vi "HEWH Spec Data.vi"(5 "Water Heater Type":T7, 7 "Test Type":T1, 8 "error in (no error)":errorcluster, 11 "UEF Calculated Values Input":T2 {"Data Indexes"."15 sec after Draw Index" format="%#.2f"; "Data Indexes"."15 sec after Draw Timestamp" format="%#.2f"; "Data Indexes"."Test Start Timestamp" format="%.2f"; "Data Indexes"."Test End Timestamp" format="%.2f"; "Data Indexes"."T0 Timestamp" format="%.2f"; "Data Indexes"."Tsf Timestamp" format="%.2f"; "Data Indexes"."Tsu0 Timestamp" format="%.2f"; "Data Indexes"."Tmax1 Timestamp" format="%.2f"; "Data Indexes"."Draw Index Timestamp" format="%#.2f"; "Data Indexes"."Non-Draw Timestamp" format="%#.2f"; "Data Indexes"."Heating Timestamp" format="%#.2f"; "Data Indexes"."Start Energy (BTU-Gas)" format="%.6f"; "Data Indexes"."Start Watt Hours" format="%.6f"; "Static Data"."V - Volume of Wh (True)" format="%.5f"; "Static Data"."T-Ambinet Nominal (°F)" format="%.5f"; "Static Data"."T-Inlet Setpoint (°F)" format="%.5f"; "Static Data"."T-Wh Setpoint (°F)" format="%.5f"; "Sampled Data"."Qe (Wh)" format="%.5f"; "Sampled Data"."Tau stby2 (hr)" format="%.5f"; "Sampled Data"."Tastby2 (°F)" format="%.5f"; "Sampled Data"."Qf (BTU)" format="%.5f"; "Sampled Data"."Qe (BTU)" format="%.5f"; "Sampled Data"."Tmax1 (°F)" format="%.5f"; "Sampled Data"."T0 (°F)" format="%.5f"; "Sampled Data"."Qr (BTU)" format="%.5f"; "Sampled Data"."T 24(°F)" format="%.5f"; "Sampled Data"."T astby(°F)" format="%.5f"; "Sampled Data"."T tstby(°F)" format="%.5f"; "Sampled Data"."T su0(°F)" format="%.5f"; "Sampled Data"."T suf(°F)" format="%.5f"; "Sampled Data"."Tau stby_1 (hr)" format="%.5f"; "Sampled Data"."Qsuf (BTU)" format="%.5f"; "Sampled Data"."Qsu0 (BTU)" format="%.5f"; "Calculated Values"."Draw Bonus Volume (gal)" format="%.6f"; "Calculated Values"."Adjustment Factor" format="%.6f"; "Calculated Values"."T*avg_del(n-1)" format="%.6f"; "Calculated Values"."T*min(n-1)" format="%.6f"; "Calculated Values"."T*avg_del(n)" format="%.6f"; "Calculated Values"."Vn" format="%.6f"; "Calculated Values"."Qdm (BTU)" format="%.6f"; "Calculated Values"."QHWD (BTU)" format="%.6f"; "Calculated Values"."QHW (BTU)" format="%.6f"; "Calculated Values"."UEF" format="%.6f"; "Calculated Values"."QHW67 (BTU)" format="%.6f"; "Calculated Values"."Qda (BTU)" format="%.6f"; "Calculated Values"."Qd (BTU)" format="%.6f"; "Calculated Values"."Q (BTU)" format="%.6f"; "Calculated Values"."UA (BTU/(hr*F))" format="%.6f"; "Calculated Values"."Qhr (BTU/hr)" format="%.6f"; "Calculated Values"."Qstby (BTU)" format="%.6f"; "Calculated Values"."nu_r" format="%.6f"; "Calculated Values"."CpUEF (BTU/(lb*F))" format="%.6f"; "Calculated Values"."rho_nu (lb/gal)" format="%.6f"; "Calculated Values"."V1- Vol (Gal)" format="%.6f"; "Calculated Values"."M cluster mass removed (lb)" format="%.6f"; "Calculated Values"."Cp theoretical (BTU/(lbm °F))" format="%.6f"; "Calculated Values"."Tin1 - Mean Inlet 1st Cluster (°F)" format="%.6f"; "Calculated Values"."Tdel1-Mean Outlet 1st Cluster(°F)" format="%.6f"; "Calculated Values"."Cp 24 (BTU/(lb*F))" format="%.6f"; "Calculated Values"."Cp standby (BTU/(lb*F))" format="%.6f"; "Calculated Values"."Cp2 (BTU/(lb*F))" format="%.6f"; "Calculated Values"."Cp1 (BTU/(lb*F))" format="%.6f"; "Calculated Values"."rho 24 (lb/gal)" format="%.6f"; "Calculated Values"."rho standby (lb/gal)" format="%.6f"; "Calculated Values"."rho 2 (lb/gal)" format="%.6f"; "Calculated Values"."Density of cold water All (lbm/gal)" format="%#.3g"; "Calculated Values"."CpHW (BTU/(lbm °F))" format="%#.3g"; "Calculated Values"."Density of hot water All (lbm/gal)" format="%#.3g"; "Calculated Values"."Mass of water All (lbm)" format="%#.3f"}) -> (0 "error out":errorcluster, 3 "UEF Calculated Values Output":T2 {"Data Indexes"."15 sec after Draw Index" format="%#.2f"; "Data Indexes"."15 sec after Draw Timestamp" format="%#.2f"; "Data Indexes"."Test Start Timestamp" format="%.2f"; "Data Indexes"."Test End Timestamp" format="%.2f"; "Data Indexes"."T0 Timestamp" format="%.2f"; "Data Indexes"."Tsf Timestamp" format="%.2f"; "Data Indexes"."Tsu0 Timestamp" format="%.2f"; "Data Indexes"."Tmax1 Timestamp" format="%.2f"; "Data Indexes"."Draw Index Timestamp" format="%#.2f"; "Data Indexes"."Non-Draw Timestamp" format="%#.2f"; "Data Indexes"."Heating Timestamp" format="%#.2f"; "Data Indexes"."Start Energy (BTU-Gas)" format="%.6f"; "Data Indexes"."Start Watt Hours" format="%.6f"; "Static Data"."V - Volume of Wh (True)" format="%.5f"; "Static Data"."T-Ambinet Nominal (°F)" format="%.5f"; "Static Data"."T-Inlet Setpoint (°F)" format="%.5f"; "Static Data"."T-Wh Setpoint (°F)" format="%.5f"; "Sampled Data"."Qe (Wh)" format="%.5f"; "Sampled Data"."Tau stby2 (hr)" format="%.5f"; "Sampled Data"."Tastby2 (°F)" format="%.5f"; "Sampled Data"."Qf (BTU)" format="%.5f"; "Sampled Data"."Qe (BTU)" format="%.5f"; "Sampled Data"."Tmax1 (°F)" format="%.5f"; "Sampled Data"."T0 (°F)" format="%.5f"; "Sampled Data"."Qr (BTU)" format="%.5f"; "Sampled Data"."T 24(°F)" format="%.5f"; "Sampled Data"."T astby(°F)" format="%.5f"; "Sampled Data"."T tstby(°F)" format="%.5f"; "Sampled Data"."T su0(°F)" format="%.5f"; "Sampled Data"."T suf(°F)" format="%.5f"; "Sampled Data"."Tau stby_1 (hr)" format="%.5f"; "Sampled Data"."Qsuf (BTU)" format="%.5f"; "Sampled Data"."Qsu0 (BTU)" format="%.5f"; "Calculated Values"."Draw Bonus Volume (gal)" format="%.6f"; "Calculated Values"."Adjustment Factor" format="%.6f"; "Calculated Values"."T*avg_del(n-1)" format="%.6f"; "Calculated Values"."T*min(n-1)" format="%.6f"; "Calculated Values"."T*avg_del(n)" format="%.6f"; "Calculated Values"."Vn" format="%.6f"; "Calculated Values"."Qdm (BTU)" format="%.6f"; "Calculated Values"."QHWD (BTU)" format="%.6f"; "Calculated Values"."QHW (BTU)" format="%.6f"; "Calculated Values"."UEF" format="%.6f"; "Calculated Values"."QHW67 (BTU)" format="%.6f"; "Calculated Values"."Qda (BTU)" format="%.6f"; "Calculated Values"."Qd (BTU)" format="%.6f"; "Calculated Values"."Q (BTU)" format="%.6f"; "Calculated Values"."UA (BTU/(hr*F))" format="%.6f"; "Calculated Values"."Qhr (BTU/hr)" format="%.6f"; "Calculated Values"."Qstby (BTU)" format="%.6f"; "Calculated Values"."nu_r" format="%.6f"; "Calculated Values"."CpUEF (BTU/(lb*F))" format="%.6f"; "Calculated Values"."rho_nu (lb/gal)" format="%.6f"; "Calculated Values"."V1- Vol (Gal)" format="%.6f"; "Calculated Values"."M cluster mass removed (lb)" format="%.6f"; "Calculated Values"."Cp theoretical (BTU/(lbm °F))" format="%.6f"; "Calculated Values"."Tin1 - Mean Inlet 1st Cluster (°F)" format="%.6f"; "Calculated Values"."Tdel1-Mean Outlet 1st Cluster(°F)" format="%.6f"; "Calculated Values"."Cp 24 (BTU/(lb*F))" format="%.6f"; "Calculated Values"."Cp standby (BTU/(lb*F))" format="%.6f"; "Calculated Values"."Cp2 (BTU/(lb*F))" format="%.6f"; "Calculated Values"."Cp1 (BTU/(lb*F))" format="%.6f"; "Calculated Values"."rho 24 (lb/gal)" format="%.6f"; "Calculated Values"."rho standby (lb/gal)" format="%.6f"; "Calculated Values"."rho 2 (lb/gal)" format="%.6f"; "Calculated Values"."Density of cold water All (lbm/gal)" format="%#.3g"; "Calculated Values"."CpHW (BTU/(lbm °F))" format="%#.3g"; "Calculated Values"."Density of hot water All (lbm/gal)" format="%#.3g"; "Calculated Values"."Mass of water All (lbm)" format="%#.3f"})   [LabVIEW 2023]
uses:
  Type Definitions/HEWH Water Heater Type.ctl
  Type Definitions/UEF Constants.ctl
  Type Definitions/HEWH Draw Stats.ctl
  Type Definitions/HEWH FHR Draw Type.ctl
  Type Definitions/FHR Bins.ctl
  Type Definitions/HEWH Meter Type.ctl
  Type Definitions/HEWH Test Type.ctl
panel:
  # "FHR"
  # "FHR"
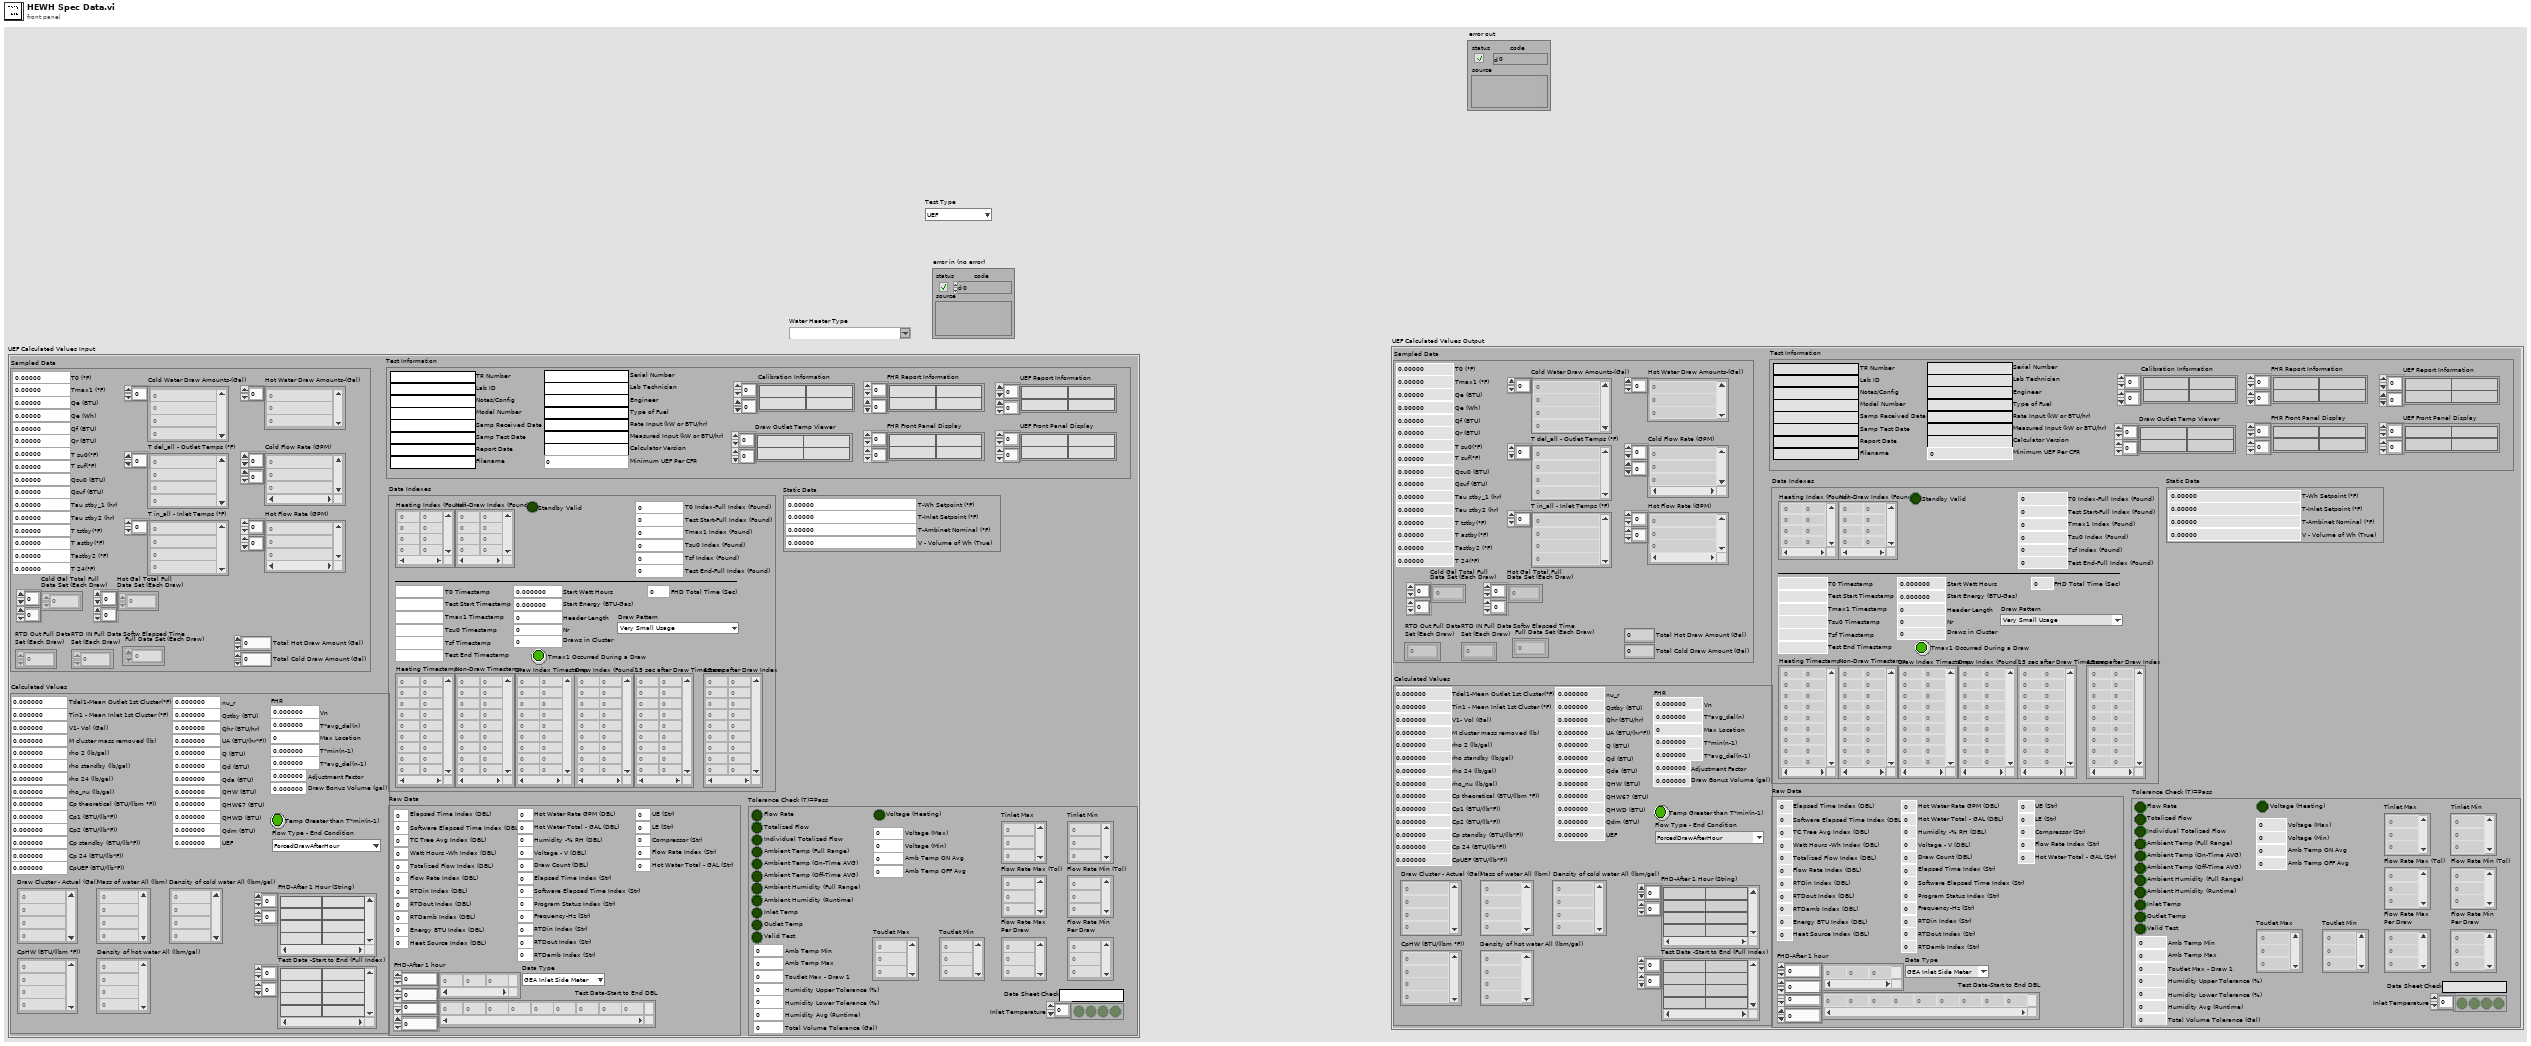
[diagram p1: front panel]
types:
  T1 = typedef "HEWH Test Type.ctl" = enum16{"UEF", "FHD"}
  T2 = typedef "UEF Constants.ctl" = cluster{"Calculated Values":T3, "Sampled Data":cluster{"Cold Water Draw Amounts-(Gal)":dbl[], "T del_all - Outlet Temps (°F)":dbl[], "T in_all - Inlet Temps (°F)":dbl[], "Qsu0 (BTU)":dbl, "Qsuf (BTU)":dbl, "Tau stby_1 (hr)":dbl, "T suf(°F)":dbl, "T su0(°F)":dbl, "T tstby(°F)":dbl, "T astby(°F)":dbl, "T 24(°F)":dbl, "Qr (BTU)":dbl, "T0 (°F)":dbl, "Tmax1 (°F)":dbl, "Qe (BTU)":dbl, "Qf (BTU)":dbl, "Tastby2 (°F)":dbl, "RTD Out Full Data\nSet (Each Draw)":dbl[][], "RTD IN Full Data\nSet (Each Draw)":dbl[][], "Tau stby2 (hr)":dbl, "Hot Water Draw Amounts-(Gal)":dbl[], "Cold Flow Rate (GPM)":dbl[][], "Hot Flow Rate (GPM)":dbl[][], "Softw Elapsed Time\n Full Data Set (Each Draw)":dbl[][], "Cold Gal Total Full\nData Set (Each Draw)":dbl[][], "Total Hot Draw Amount (Gal) ":dbl, "Total Cold Draw Amount (Gal)":dbl, "Qe (Wh)":dbl, "Hot Gal Total Full\nData Set (Each Draw)":dbl[][]}, "Static Data":cluster{"T-Wh Setpoint (°F)":dbl, "T-Inlet Setpoint (°F)":dbl, "T-Ambinet Nominal (°F)":dbl, "V - Volume of Wh (True)":dbl}, "Data Indexes":cluster{"Test Start-Full Index (Found)":i32, "Header Length":i32, "Draw Index (Found)":i32[][], "Nr":i32, "Start Watt Hours":dbl, "Tsu0 Index (Found)":i32, "Tsf Index (Found)":i32, "Start Energy (BTU-Gas)":dbl, "Draws in Cluster":i32, "T0 Index-Full Index (Found)":i32, "Non-Draw Index (Found)":i32[][], "Tmax1 Index (Found)":i32, "Test End-Full Index (Found)":i32, "Heating Index (Found)":i32[][], "Heating Timestamp":dbl[][], "Non-Draw Timestamp":dbl[][], "Draw Index Timestamp":dbl[][], "Tmax1 Timestamp":dbl, "Tsu0 Timestamp":dbl, "Tsf Timestamp":dbl, "T0 Timestamp":dbl, "Test End Timestamp":dbl, "Test Start Timestamp":dbl, "15 sec after Draw Timestamp":dbl[][], "15 sec after Draw Index":dbl[][], "Tmax1 Occurred During a Draw":bool, "FHD Total Time (Sec)":dbl, "Draw Pattern":T5, "Standby Valid":bool}, "Raw Data":cluster{"Elapsed Time Index (DBL)":i32, "Software Elapsed Time Index (DBL)":i32, "TC Tree Avg Index (DBL)":i32, "Watt Hours -Wh Index (DBL)":i32, "Energy BTU Index (DBL)":i32, "Totalized Flow Index (DBL)":i32, "Flow Rate Index (DBL)":i32, "Program Status Index (Str)":i32, "RTDin Index (DBL)":i32, "RTDout Index (DBL)":i32, "RTDamb Index (DBL)":i32, "Test Data-Start to End DBL":dbl[][], "Data Type":T6, "Heat Source Index (DBL)":i32, "Hot Water Rate GPM (DBL)":i32, "Hot Water Total - GAL (DBL)":i32, "FHD-After 1 hour":dbl[][], "Humidity -% RH (DBL)":i32, "Voltage - V (DBL)":i32, "Draw Count (DBL)":i32, "Elapsed Time Index (Str)":i32, "Software Elapsed Time Index (Str)":i32, "Frequency-Hz (Str)":i32, "RTDin Index (Str)":i32, "RTDout Index (Str)":i32, "RTDamb Index (Str)":i32, "UE (Str)":i32, "LE (Str)":i32, "Compressor (Str)":i32, "Flow Rate Index (Str)":i32, "Hot Water Total - GAL (Str)":i32}, "Tolerance Check (T)=Pass":cluster{"Flow Rate":bool, "Totalized Flow":bool, "Ambient Temp (Full Range)":bool, "Ambient Humidity (Full Range)":bool, "Inlet Temp":bool, "Outlet Temp":bool, "Valid Test":bool, "Individual Totalized Flow":bool, "Data Sheet Check":string, "Inlet Temperature":bool[], "Tinlet Max":dbl[], "Tinlet Min":dbl[], "Flow Rate Max (Tol)":dbl[], "Flow Rate Min (Tol)":dbl[], "Amb Temp Max":dbl, "Amb Temp Min":dbl, "Toutlet Max - Draw 1":dbl, "Humidity Upper Tolerance (%)":dbl, "Total Volume Tolerance (Gal)":dbl, "Humidity Lower Tolerance (%)":dbl, "Flow Rate Max\nPer Draw":dbl[], "Flow Rate Min\nPer Draw":dbl[], "Ambient Humidity (Runtime)":bool, "Humidity Avg (Runtime)":dbl, "Ambient Temp (On-Time AVG)":bool, "Ambient Temp (Off-Time AVG)":bool, "Amb Temp OFF Avg":dbl, "Amb Temp ON Avg":dbl, "Voltage (Heating)":bool, "Voltage (Min)":dbl, "Voltage (Max)":dbl, "Toutlet Max":dbl[], "Toutlet Min":dbl[]}, "Test Information":cluster{"TR Number":string, "Lab ID":string, "Notes/Config":string, "Model Number":string, "Serial Number":string, "Lab Technician":string, "Engineer":string, "Type of Fuel":string, "Samp Received Date":string, "Samp Test Date":string, "Report Date":string, "Rate Input (kW or BTU/hr)":string, "Measured Input (kW or BTU/hr)":string, "Filename":string, "Calibration Information":string[][], "Calculator Version":string, "Minimum UEF Per CFR":dbl, "UEF Report Information":string[][], "FHR Report Information":string[][], "FHR Front Panel Display":string[][], "UEF Front Panel Display":string[][], "Draw Outlet Temp Viewer":string[][]}}
  T3 = typedef "HEWH Draw Stats.ctl" = cluster{"Draw Cluster - Actual (Gal)":dbl[], "Mass of water All (lbm)":dbl[], "Density of hot water All (lbm/gal)":dbl[], "CpHW (BTU/(lbm °F))":dbl[], "rho 2 (lb/gal)":dbl, "rho standby (lb/gal)":dbl, "rho 24 (lb/gal)":dbl, "Cp1 (BTU/(lb*F))":dbl, "Cp2 (BTU/(lb*F))":dbl, "Cp standby (BTU/(lb*F))":dbl, "Cp 24 (BTU/(lb*F))":dbl, "nu_r":dbl, "Qstby (BTU)":dbl, "Qhr (BTU/hr)":dbl, "UA (BTU/(hr*F))":dbl, "Q (BTU)":dbl, "Qd (BTU)":dbl, "Qda (BTU)":dbl, "QHW67 (BTU)":dbl, "UEF":dbl, "Tdel1-Mean Outlet 1st Cluster(°F)":dbl, "Tin1 - Mean Inlet 1st Cluster (°F)":dbl, "Cp theoretical (BTU/(lbm °F))":dbl, "M cluster mass removed (lb)":dbl, "V1- Vol (Gal)":dbl, "Test Data -Start to End (Full Index)":string[][], "rho_nu (lb/gal)":dbl, "Density of cold water All (lbm/gal)":dbl[], "CpUEF (BTU/(lb*F))":dbl, "QHW (BTU)":dbl, "QHWD (BTU)":dbl, "Qdm (BTU)":dbl, "FHD-After 1 Hour (String)":string[][], "Vn":dbl, "T*avg_del(n)":dbl, "Max Location":i32, "T*min(n-1)":dbl, "T*avg_del(n-1)":dbl, "Temp Greater than T*min(n-1)":bool, "Adjustment Factor":dbl, "Draw Bonus Volume (gal)":dbl, "Flow Type - End Condition":T4}
  T4 = typedef "HEWH FHR Draw Type.ctl" = enum16{"ForcedDrawAfterHour", "HeatingCutoffBeforeHour"}
  T5 = typedef "FHR Bins.ctl" = enum16{"Very Small Usage", "Low Usage", "Medium Usage", "High Usage", "Undefined"}
  T6 = typedef "HEWH Meter Type.ctl" = enum16{"GEA Inlet Side Meter", "GEA Outlet Side Meter", "CSA Inlet Side Meter"}
  T7 = typedef "HEWH Water Heater Type.ctl" = string
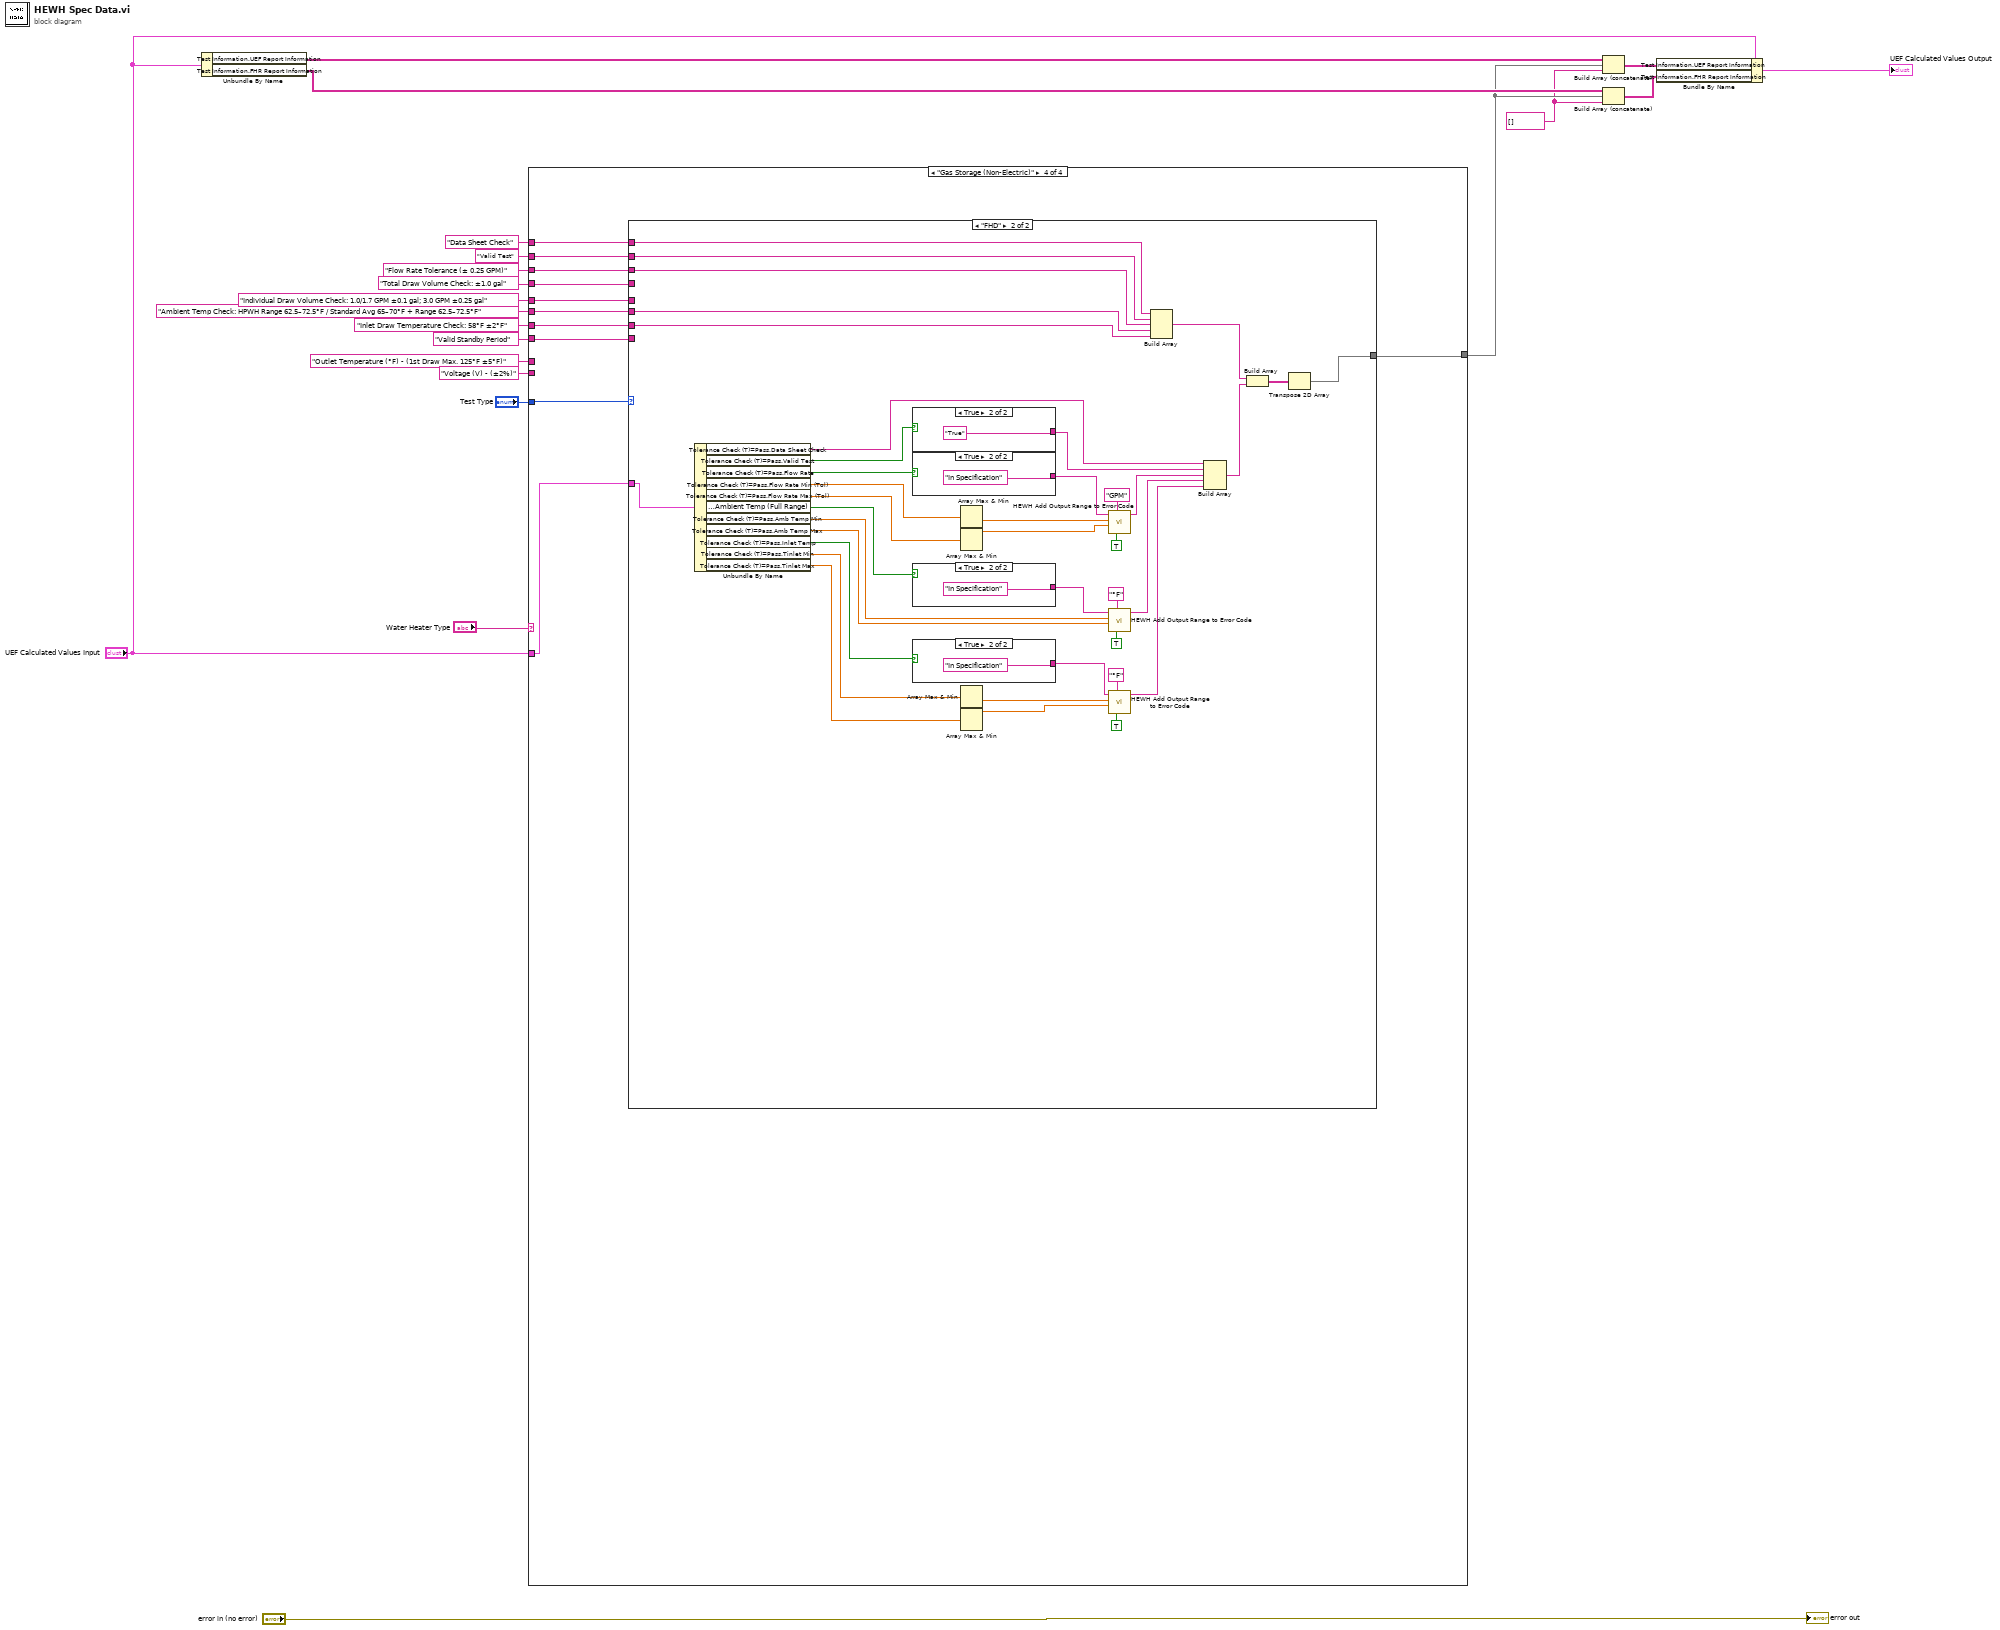
[diagram p0: block diagram]
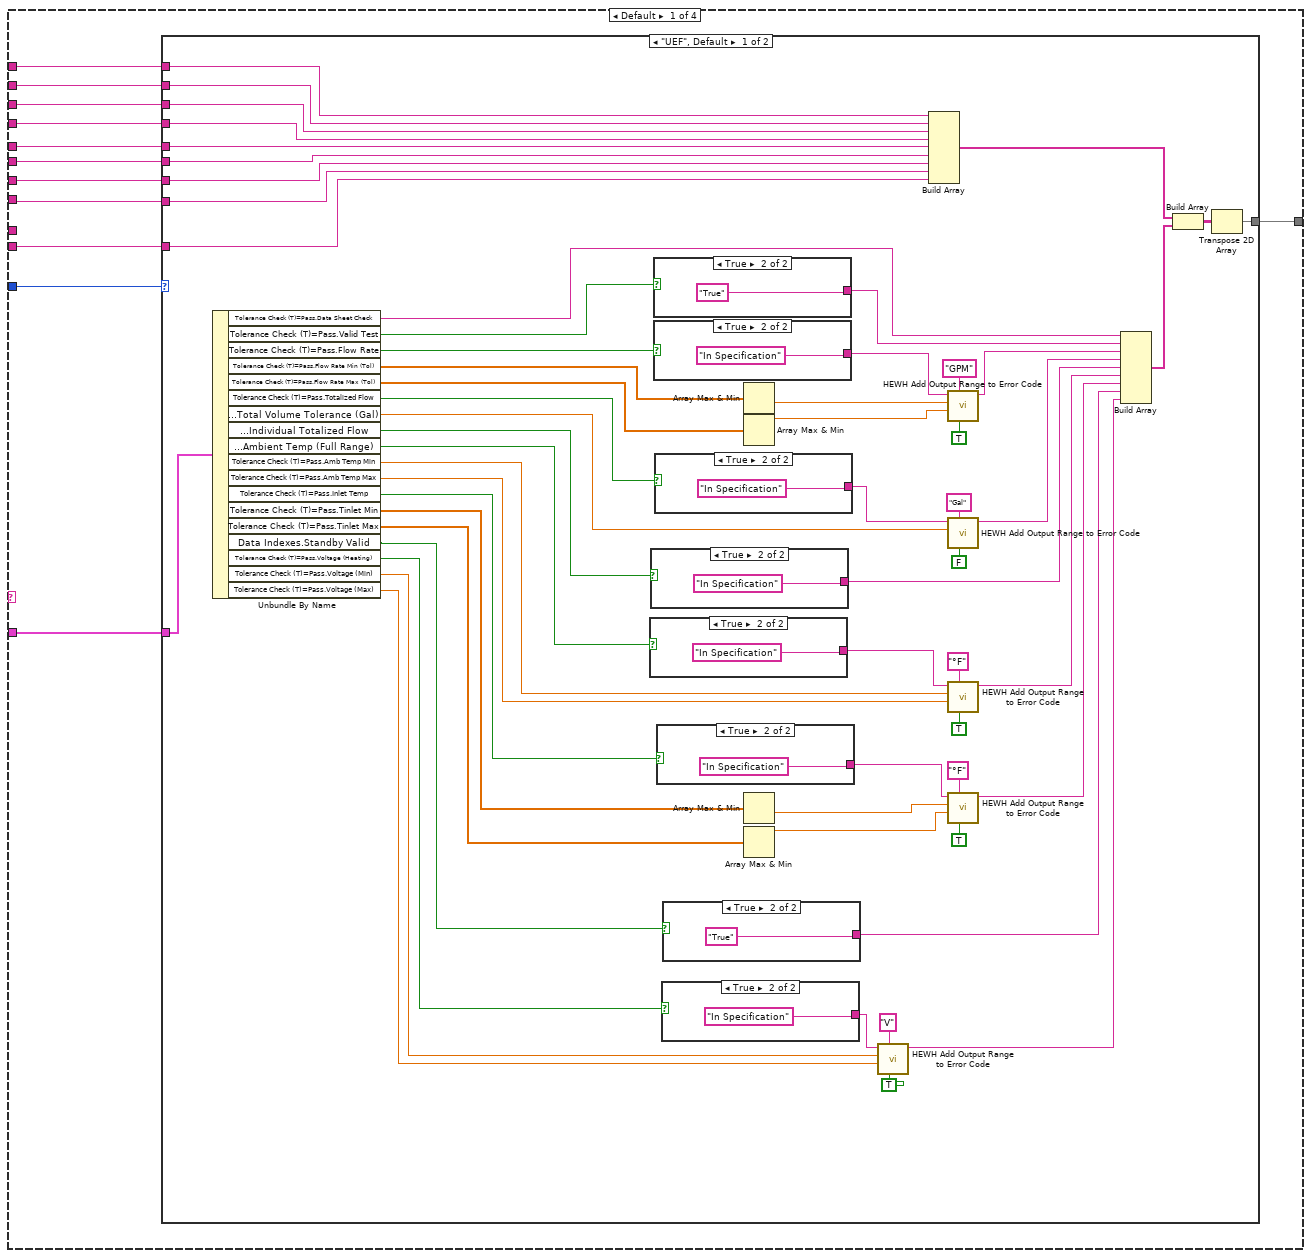
[diagram p2: hidden frame]
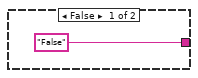
[diagram p3: hidden frame]
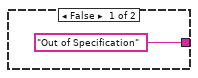
[diagram p4: hidden frame]
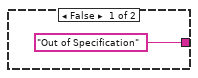
[diagram p5: hidden frame]
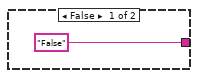
[diagram p6: hidden frame]
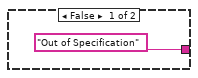
[diagram p7: hidden frame]
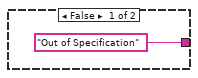
[diagram p8: hidden frame]
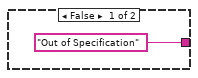
[diagram p9: hidden frame]
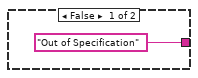
[diagram p10: hidden frame]
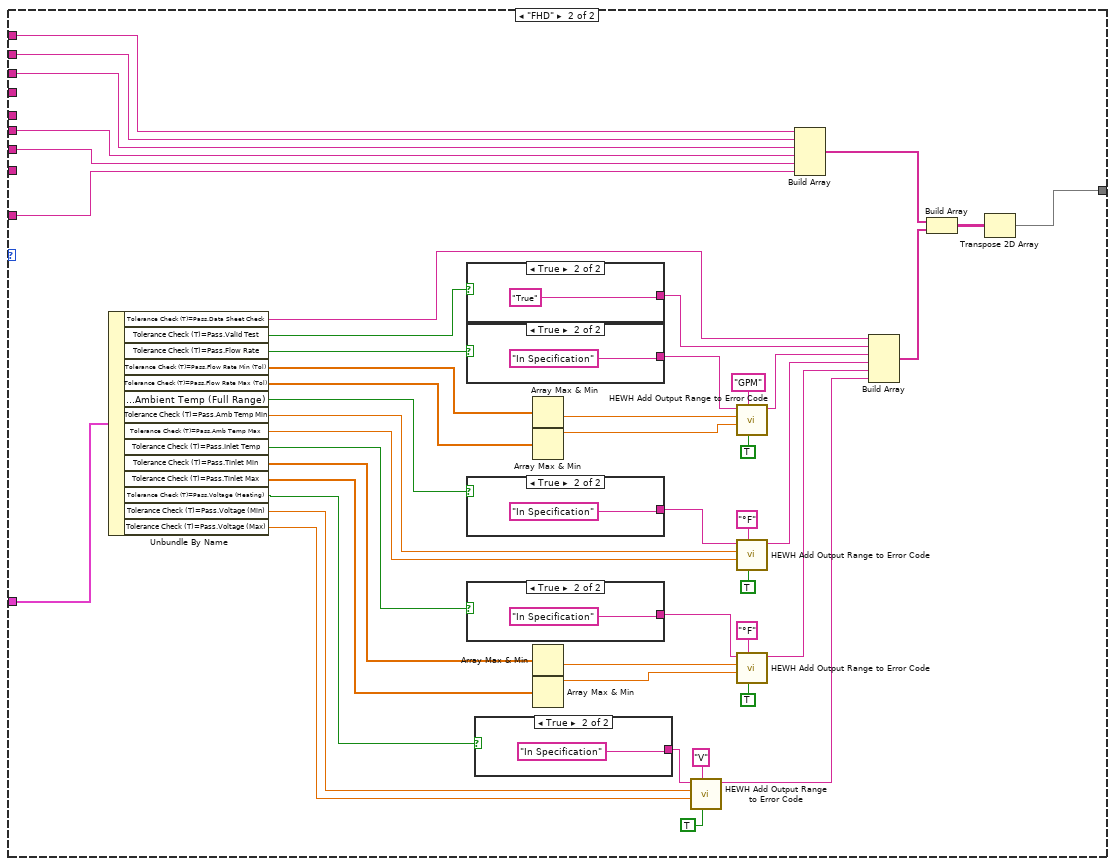
[diagram p11: hidden frame]
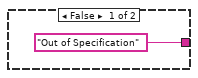
[diagram p12: hidden frame]
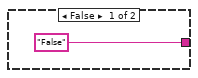
[diagram p13: hidden frame]
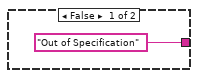
[diagram p14: hidden frame]
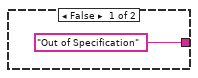
[diagram p15: hidden frame]
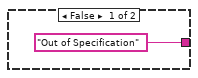
[diagram p16: hidden frame]
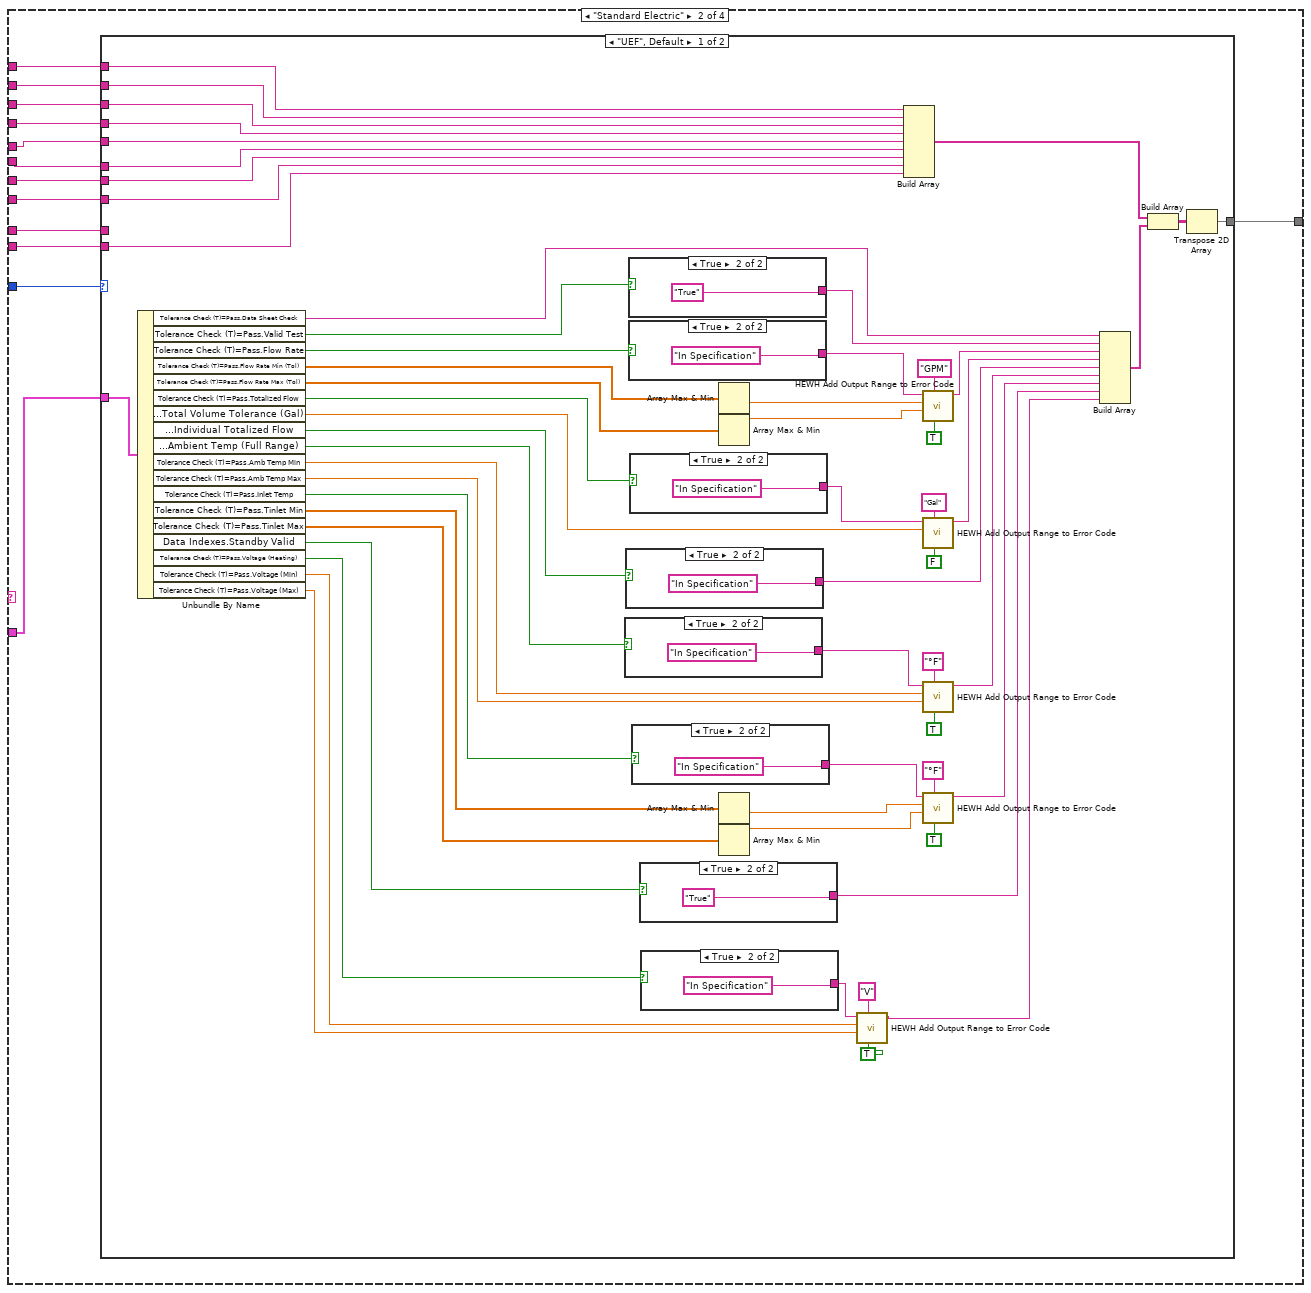
[diagram p17: hidden frame]
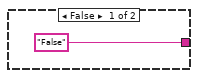
[diagram p18: hidden frame]
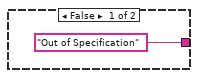
[diagram p19: hidden frame]
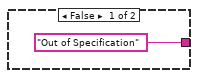
[diagram p20: hidden frame]
diagram:
  w4 = string[] []
  n1 = Unbundle By Name("UEF Calculated Values Input") -> ("Test Information.UEF Report Information"=w8:string[][], "Test Information.FHR Report Information"=w7:string[][])
  n2 = case shown="\"Gas Storage (Non-Electric)\"" "Water Heater Type" {
    tunnel: "UEF Calculated Values Input" -> [w33 w177 w328 w544]
    tunnel: [w32 w176 w327 w543] -> w5
    tunnel: "Test Type" -> [w31 w175 w326 w542]
    tunnel: "Voltage (V) - (±2%)" -> [w30 w169 w319 _]
    tunnel: "Inlet Draw Temperature Check: 58°F ±2°F" -> [w29 w170 w320 w535]
    tunnel: "Ambient Temp Check: HPWH Range 62.5–72.5°F / Standard Avg 65–70°F + Range 62.5–72.5°F" -> [w28 w171 _ w536]
    tunnel: "Individual Draw Volume Check: 1.0/1.7 GPM ±0.1 gal; 3.0 GPM ±0.25 gal" -> [w27 w166 w321 w537]
    tunnel: "Total Draw Volume Check: ±1.0 gal" -> [w26 w167 w322 w538]
    tunnel: "Flow Rate Tolerance (± 0.25 GPM)" -> [w25 w172 w323 w539]
    tunnel: "Valid Test" -> [w24 w173 w324 w540]
    tunnel: "Data Sheet Check" -> [w23 w174 w325 w541]
    tunnel: "Outlet Temperature (°F) - (1st Draw Max. 125°F ±5°F)" -> [_ w168 _ _]
    tunnel: "Valid Standby Period" -> [w22 w165 w318 w534]
    frame Default {
      n3 = case shown="\"UEF\", Default" w31 {
        tunnel: w33 -> [w92 w145]
        tunnel: [w84 w144] -> w32
        tunnel: w23 -> [w44 w114]
        tunnel: w24 -> [w43 w113]
        tunnel: w25 -> [w42 w112]
        tunnel: w26 -> [w41 _]
        tunnel: w27 -> [w40 _]
        tunnel: w28 -> [w39 w111]
        tunnel: w29 -> [w37 w110]
        tunnel: w30 -> [w38 w109]
        tunnel: w22 -> [w34 _]
        frame "UEF", Default {
          n4 = Unbundle By Name(w92) -> ("Tolerance Check (T)=Pass.Data Sheet Check"=w81:string, "Tolerance Check (T)=Pass.Valid Test"=w83:bool, "Tolerance Check (T)=Pass.Flow Rate"=w91:bool, "Tolerance Check (T)=Pass.Flow Rate Min (Tol)"=w58:dbl[], "Tolerance Check (T)=Pass.Flow Rate Max (Tol)"=w57:dbl[], "Tolerance Check (T)=Pass.Totalized Flow"=w90:bool, "Tolerance Check (T)=Pass.Total Volume Tolerance (Gal)"=w52:dbl, "Tolerance Check (T)=Pass.Individual Totalized Flow"=w79:bool, "Tolerance Check (T)=Pass.Ambient Temp (Full Range)"=w89:bool, "Tolerance Check (T)=Pass.Amb Temp Min"=w74:dbl, "Tolerance Check (T)=Pass.Amb Temp Max"=w73:dbl, "Tolerance Check (T)=Pass.Inlet Temp"=w88:bool, "Tolerance Check (T)=Pass.Tinlet Min"=w68:dbl[], "Tolerance Check (T)=Pass.Tinlet Max"=w67:dbl[], "Data Indexes.Standby Valid"=w36:bool, "Tolerance Check (T)=Pass.Voltage (Heating)"=w47:bool, "Tolerance Check (T)=Pass.Voltage (Min)"=w46:dbl, "Tolerance Check (T)=Pass.Voltage (Max)"=w45:dbl)
          n5 = case shown="True" w89 {
            tunnel: ["Out of Specification" "In Specification"] -> w76
            frame False {
            }
            frame True {
            }
          }
          n6 = case shown="True" w79 {
            tunnel: ["Out of Specification" "In Specification"] -> w80
            frame False {
            }
            frame True {
            }
          }
          n7 = case shown="True" w83 {
            tunnel: ["False" "True"] -> w82
            frame False {
            }
            frame True {
            }
          }
          n8 = case shown="True" w91 {
            tunnel: ["Out of Specification" "In Specification"] -> w60
            frame False {
            }
            frame True {
            }
          }
          n9 = case shown="True" w90 {
            tunnel: ["Out of Specification" "In Specification"] -> w54
            frame False {
            }
            frame True {
            }
          }
          n10 = case shown="True" w88 {
            tunnel: ["Out of Specification" "In Specification"] -> w66
            frame False {
            }
            frame True {
            }
          }
          n11 = case shown="True" w47 {
            tunnel: ["Out of Specification" "In Specification"] -> w51
            frame False {
            }
            frame True {
            }
          }
          n12 = case shown="True" w36 {
            tunnel: ["False" "True"] -> w35
            frame False {
            }
            frame True {
            }
          }
          n13 = Array Max & Min(array=w58) -> (min value=w64:dbl)  [unwired: 3 out]
          n14 = Array Max & Min(array=w57) -> (max value=w63:dbl)  [unwired: 3 out]
          n15 = Array Max & Min(array=w68) -> (min value=w72:dbl)  [unwired: 3 out]
          n16 = Array Max & Min(array=w67) -> (max value=w71:dbl)  [unwired: 3 out]
          n17 = call "HEWH Add Output Range to Error Code.vi"("Range?"=TRUE, "Units"="V", "Value Max"=w45, "Value Min"=w46, "Input String"=w51) -> ("Display Range"=w48:string)  [unwired: 6 in]
          n18 = Build Array(w44, w43, w42, w41, w40, w39, w37, w34, w38) -> (w87:string[])
          n19 = call "HEWH Add Output Range to Error Code.vi"("Range?"=TRUE, "Units"="GPM", "Value Max"=w63, "Value Min"=w64, "Input String"=w60) -> ("Display Range"=w59:string)  [unwired: 6 in]
          n20 = call "HEWH Add Output Range to Error Code.vi"("Range?"=FALSE, "Units"="Gal", "Value Min"=w52, "Input String"=w54) -> ("Display Range"=w53:string)  [unwired: 7 in]
          n21 = call "HEWH Add Output Range to Error Code.vi"("Range?"=TRUE, "Units"="°F", "Value Max"=w73, "Value Min"=w74, "Input String"=w76) -> ("Display Range"=w75:string)  [unwired: 6 in]
          n22 = call "HEWH Add Output Range to Error Code.vi"("Range?"=TRUE, "Units"="°F", "Value Max"=w71, "Value Min"=w72, "Input String"=w66) -> ("Display Range"=w65:string)  [unwired: 6 in]
          n23 = Build Array(w81, w82, w59, w53, w80, w75, w65, w35, w48) -> (w86:string[])
          n24 = Build Array(w87, w86) -> (w85:string[][])
          n25 = Transpose 2D Array(2D array=w85) -> (transposed array=w84:string[][])
        }
        frame "FHD" {
          n26 = Unbundle By Name(w145) -> ("Tolerance Check (T)=Pass.Data Sheet Check"=w146:string, "Tolerance Check (T)=Pass.Valid Test"=w148:bool, "Tolerance Check (T)=Pass.Flow Rate"=w154:bool, "Tolerance Check (T)=Pass.Flow Rate Min (Tol)"=w125:dbl[], "Tolerance Check (T)=Pass.Flow Rate Max (Tol)"=w124:dbl[], "Tolerance Check (T)=Pass.Ambient Temp (Full Range)"=w153:bool, "Tolerance Check (T)=Pass.Amb Temp Min"=w139:dbl, "Tolerance Check (T)=Pass.Amb Temp Max"=w138:dbl, "Tolerance Check (T)=Pass.Inlet Temp"=w152:bool, "Tolerance Check (T)=Pass.Tinlet Min"=w131:dbl[], "Tolerance Check (T)=Pass.Tinlet Max"=w130:dbl[], "Tolerance Check (T)=Pass.Voltage (Heating)"=w118:bool, "Tolerance Check (T)=Pass.Voltage (Min)"=w117:dbl, "Tolerance Check (T)=Pass.Voltage (Max)"=w116:dbl)
          n27 = case shown="True" w148 {
            tunnel: ["False" "True"] -> w147
            frame False {
            }
            frame True {
            }
          }
          n28 = case shown="True" w154 {
            tunnel: ["Out of Specification" "In Specification"] -> w123
            frame False {
            }
            frame True {
            }
          }
          n29 = case shown="True" w153 {
            tunnel: ["Out of Specification" "In Specification"] -> w141
            frame False {
            }
            frame True {
            }
          }
          n30 = case shown="True" w152 {
            tunnel: ["Out of Specification" "In Specification"] -> w133
            frame False {
            }
            frame True {
            }
          }
          n31 = case shown="True" w118 {
            tunnel: ["Out of Specification" "In Specification"] -> w121
            frame False {
            }
            frame True {
            }
          }
          n32 = Array Max & Min(array=w125) -> (min value=w129:dbl)  [unwired: 3 out]
          n33 = Array Max & Min(array=w124) -> (max value=w128:dbl)  [unwired: 3 out]
          n34 = Array Max & Min(array=w131) -> (min value=w137:dbl)  [unwired: 3 out]
          n35 = Array Max & Min(array=w130) -> (max value=w136:dbl)  [unwired: 3 out]
          n36 = call "HEWH Add Output Range to Error Code.vi"("Range?"=TRUE, "Units"="V", "Value Max"=w116, "Value Min"=w117, "Input String"=w121) -> ("Display Range"=w115:string)  [unwired: 6 in]
          n37 = call "HEWH Add Output Range to Error Code.vi"("Range?"=TRUE, "Units"="GPM", "Value Max"=w128, "Value Min"=w129, "Input String"=w123) -> ("Display Range"=w122:string)  [unwired: 6 in]
          n38 = call "HEWH Add Output Range to Error Code.vi"("Range?"=TRUE, "Units"="°F", "Value Max"=w138, "Value Min"=w139, "Input String"=w141) -> ("Display Range"=w140:string)  [unwired: 6 in]
          n39 = call "HEWH Add Output Range to Error Code.vi"("Range?"=TRUE, "Units"="°F", "Value Max"=w136, "Value Min"=w137, "Input String"=w133) -> ("Display Range"=w132:string)  [unwired: 6 in]
          n40 = Build Array(w114, w113, w112, w111, w110, w109) -> (w151:string[])
          n41 = Build Array(w146, w147, w122, w140, w132, w115) -> (w150:string[])
          n42 = Build Array(w151, w150) -> (w149:string[][])
          n43 = Transpose 2D Array(2D array=w149) -> (transposed array=w144:string[][])
        }
      }
    }
    frame "Standard Electric" {
      n44 = case shown="\"UEF\", Default" w175 {
        tunnel: w177 -> [w236 w296]
        tunnel: [w228 w295] -> w176
        tunnel: w174 -> [w188 w259]
        tunnel: w173 -> [w187 w258]
        tunnel: w172 -> [w186 w257]
        tunnel: w171 -> [w183 w256]
        tunnel: w170 -> [w182 w255]
        tunnel: w169 -> [w181 w254]
        tunnel: w168 -> [_ w253]
        tunnel: w167 -> [w185 _]
        tunnel: w166 -> [w184 _]
        tunnel: w165 -> [w180 _]
        frame "UEF", Default {
          n45 = Unbundle By Name(w236) -> ("Tolerance Check (T)=Pass.Data Sheet Check"=w225:string, "Tolerance Check (T)=Pass.Valid Test"=w227:bool, "Tolerance Check (T)=Pass.Flow Rate"=w235:bool, "Tolerance Check (T)=Pass.Flow Rate Min (Tol)"=w202:dbl[], "Tolerance Check (T)=Pass.Flow Rate Max (Tol)"=w201:dbl[], "Tolerance Check (T)=Pass.Totalized Flow"=w234:bool, "Tolerance Check (T)=Pass.Total Volume Tolerance (Gal)"=w196:dbl, "Tolerance Check (T)=Pass.Individual Totalized Flow"=w223:bool, "Tolerance Check (T)=Pass.Ambient Temp (Full Range)"=w233:bool, "Tolerance Check (T)=Pass.Amb Temp Min"=w218:dbl, "Tolerance Check (T)=Pass.Amb Temp Max"=w217:dbl, "Tolerance Check (T)=Pass.Inlet Temp"=w232:bool, "Tolerance Check (T)=Pass.Tinlet Min"=w212:dbl[], "Tolerance Check (T)=Pass.Tinlet Max"=w211:dbl[], "Data Indexes.Standby Valid"=w179:bool, "Tolerance Check (T)=Pass.Voltage (Heating)"=w192:bool, "Tolerance Check (T)=Pass.Voltage (Min)"=w191:dbl, "Tolerance Check (T)=Pass.Voltage (Max)"=w190:dbl)
          n46 = case shown="True" w233 {
            tunnel: ["Out of Specification" "In Specification"] -> w220
            frame False {
            }
            frame True {
            }
          }
          n47 = case shown="True" w223 {
            tunnel: ["Out of Specification" "In Specification"] -> w224
            frame False {
            }
            frame True {
            }
          }
          n48 = case shown="True" w227 {
            tunnel: ["False" "True"] -> w226
            frame False {
            }
            frame True {
            }
          }
          n49 = case shown="True" w235 {
            tunnel: ["Out of Specification" "In Specification"] -> w204
            frame False {
            }
            frame True {
            }
          }
          n50 = case shown="True" w234 {
            tunnel: ["Out of Specification" "In Specification"] -> w198
            frame False {
            }
            frame True {
            }
          }
          n51 = case shown="True" w232 {
            tunnel: ["Out of Specification" "In Specification"] -> w210
            frame False {
            }
            frame True {
            }
          }
          n52 = case shown="True" w179 {
            tunnel: ["False" "True"] -> w178
            frame False {
            }
            frame True {
            }
          }
          n53 = case shown="True" w192 {
            tunnel: ["Out of Specification" "In Specification"] -> w195
            frame False {
            }
            frame True {
            }
          }
          n54 = Array Max & Min(array=w202) -> (min value=w208:dbl)  [unwired: 3 out]
          n55 = Array Max & Min(array=w201) -> (max value=w207:dbl)  [unwired: 3 out]
          n56 = Array Max & Min(array=w212) -> (min value=w216:dbl)  [unwired: 3 out]
          n57 = Array Max & Min(array=w211) -> (max value=w215:dbl)  [unwired: 3 out]
          n58 = call "HEWH Add Output Range to Error Code.vi"("Range?"=TRUE, "Units"="V", "Value Max"=w190, "Value Min"=w191, "Input String"=w195) -> ("Display Range"=w189:string)  [unwired: 6 in]
          n59 = Build Array(w188, w187, w186, w185, w184, w183, w182, w180, w181) -> (w231:string[])
          n60 = call "HEWH Add Output Range to Error Code.vi"("Range?"=TRUE, "Units"="GPM", "Value Max"=w207, "Value Min"=w208, "Input String"=w204) -> ("Display Range"=w203:string)  [unwired: 6 in]
          n61 = call "HEWH Add Output Range to Error Code.vi"("Range?"=FALSE, "Units"="Gal", "Value Min"=w196, "Input String"=w198) -> ("Display Range"=w197:string)  [unwired: 7 in]
          n62 = call "HEWH Add Output Range to Error Code.vi"("Range?"=TRUE, "Units"="°F", "Value Max"=w217, "Value Min"=w218, "Input String"=w220) -> ("Display Range"=w219:string)  [unwired: 6 in]
          n63 = call "HEWH Add Output Range to Error Code.vi"("Range?"=TRUE, "Units"="°F", "Value Max"=w215, "Value Min"=w216, "Input String"=w210) -> ("Display Range"=w209:string)  [unwired: 6 in]
          n64 = Build Array(w225, w226, w203, w197, w224, w219, w209, w178, w189) -> (w230:string[])
          n65 = Build Array(w231, w230) -> (w229:string[][])
          n66 = Transpose 2D Array(2D array=w229) -> (transposed array=w228:string[][])
        }
        frame "FHD" {
          n67 = Unbundle By Name(w296) -> ("Tolerance Check (T)=Pass.Data Sheet Check"=w297:string, "Tolerance Check (T)=Pass.Valid Test"=w299:bool, "Tolerance Check (T)=Pass.Flow Rate"=w305:bool, "Tolerance Check (T)=Pass.Flow Rate Min (Tol)"=w276:dbl[], "Tolerance Check (T)=Pass.Flow Rate Max (Tol)"=w275:dbl[], "Tolerance Check (T)=Pass.Ambient Temp (Full Range)"=w304:bool, "Tolerance Check (T)=Pass.Amb Temp Min"=w290:dbl, "Tolerance Check (T)=Pass.Amb Temp Max"=w289:dbl, "Tolerance Check (T)=Pass.Inlet Temp"=w303:bool, "Tolerance Check (T)=Pass.Tinlet Min"=w282:dbl[], "Tolerance Check (T)=Pass.Tinlet Max"=w281:dbl[], "Tolerance Check (T)=Pass.Outlet Temp"=w269:bool, "Tolerance Check (T)=Pass.Toutlet Max - Draw 1"=w268:dbl, "Tolerance Check (T)=Pass.Voltage (Heating)"=w263:bool, "Tolerance Check (T)=Pass.Voltage (Min)"=w262:dbl, "Tolerance Check (T)=Pass.Voltage (Max)"=w261:dbl)
          n68 = case shown="True" w263 {
            tunnel: ["Out of Specification" "In Specification"] -> w266
            frame False {
            }
            frame True {
            }
          }
          n69 = case shown="True" w269 {
            tunnel: ["Out of Specification" "In Specification"] -> w272
            frame False {
            }
            frame True {
            }
          }
          n70 = case shown="True" w299 {
            tunnel: ["False" "True"] -> w298
            frame False {
            }
            frame True {
            }
          }
          n71 = case shown="True" w305 {
            tunnel: ["Out of Specification" "In Specification"] -> w274
            frame False {
            }
            frame True {
            }
          }
          n72 = case shown="True" w304 {
            tunnel: ["Out of Specification" "In Specification"] -> w292
            frame False {
            }
            frame True {
            }
          }
          n73 = case shown="True" w303 {
            tunnel: ["Out of Specification" "In Specification"] -> w284
            frame False {
            }
            frame True {
            }
          }
          n74 = Array Max & Min(array=w276) -> (min value=w280:dbl)  [unwired: 3 out]
          n75 = Array Max & Min(array=w275) -> (max value=w279:dbl)  [unwired: 3 out]
          n76 = Array Max & Min(array=w282) -> (min value=w288:dbl)  [unwired: 3 out]
          n77 = Array Max & Min(array=w281) -> (max value=w287:dbl)  [unwired: 3 out]
          n78 = call "HEWH Add Output Range to Error Code.vi"("Range?"=TRUE, "Units"="V", "Value Max"=w261, "Value Min"=w262, "Input String"=w266) -> ("Display Range"=w260:string)  [unwired: 6 in]
          n79 = call "HEWH Add Output Range to Error Code.vi"("Range?"=TRUE, "Units"="GPM", "Value Max"=w279, "Value Min"=w280, "Input String"=w274) -> ("Display Range"=w273:string)  [unwired: 6 in]
          n80 = call "HEWH Add Output Range to Error Code.vi"("Range?"=TRUE, "Units"="°F", "Value Max"=w289, "Value Min"=w290, "Input String"=w292) -> ("Display Range"=w291:string)  [unwired: 6 in]
          n81 = call "HEWH Add Output Range to Error Code.vi"("Range?"=TRUE, "Units"="°F", "Value Max"=w287, "Value Min"=w288, "Input String"=w284) -> ("Display Range"=w283:string)  [unwired: 6 in]
          n82 = call "HEWH Add Output Range to Error Code.vi"("Range?"=FALSE, "Units"="°F", "Value Min"=w268, "Input String"=w272) -> ("Display Range"=w267:string)  [unwired: 7 in]
          n83 = Build Array(w259, w258, w257, w256, w255, w253, w254) -> (w302:string[])
          n84 = Build Array(w297, w298, w273, w291, w283, w267, w260) -> (w301:string[])
          n85 = Build Array(w302, w301) -> (w300:string[][])
          n86 = Transpose 2D Array(2D array=w300) -> (transposed array=w295:string[][])
        }
      }
    }
    frame "HPWH" {
      n87 = case shown="\"FHD\"" w326 {
        tunnel: w328 -> [w416 w501]
        tunnel: [w405 w500] -> w327
        tunnel: w325 -> [w338 w445]
        tunnel: w324 -> [w337 w444]
        tunnel: w323 -> [w336 w443]
        tunnel: w322 -> [w335 _]
        tunnel: w321 -> [w334 _]
        tunnel: w320 -> [w333 w442]
        tunnel: w319 -> [w332 w441]
        tunnel: w318 -> [w331 _]
        frame "UEF", Default {
          n88 = Unbundle By Name(w416) -> ("Tolerance Check (T)=Pass.Data Sheet Check"=w401:string, "Tolerance Check (T)=Pass.Valid Test"=w404:bool, "Tolerance Check (T)=Pass.Flow Rate"=w415:bool, "Tolerance Check (T)=Pass.Flow Rate Min (Tol)"=w383:dbl[], "Tolerance Check (T)=Pass.Flow Rate Max (Tol)"=w382:dbl[], "Tolerance Check (T)=Pass.Totalized Flow"=w414:bool, "Tolerance Check (T)=Pass.Total Volume Tolerance (Gal)"=w371:dbl, "Tolerance Check (T)=Pass.Individual Totalized Flow"=w402:bool, "Tolerance Check (T)=Pass.Ambient Temp (Full Range)"=w413:bool, "Tolerance Check (T)=Pass.Amb Temp Min"=w379:dbl, "Tolerance Check (T)=Pass.Amb Temp Max"=w378:dbl, "Tolerance Check (T)=Pass.Ambient Temp (On-Time AVG)"=w366:bool, "Tolerance Check (T)=Pass.Amb Temp ON Avg"=w362:dbl, "Tolerance Check (T)=Pass.Ambient Temp (Off-Time AVG)"=w358:bool, "Tolerance Check (T)=Pass.Amb Temp OFF Avg"=w357:dbl, "Tolerance Check (T)=Pass.Ambient Humidity (Full Range)"=w411:bool, "Tolerance Check (T)=Pass.Humidity Lower Tolerance (%)"=w367:dbl, "Tolerance Check (T)=Pass.Humidity Upper Tolerance (%)"=w368:dbl, "Tolerance Check (T)=Pass.Ambient Humidity (Runtime)"=w354:bool, "Tolerance Check (T)=Pass.Humidity Avg (Runtime)"=w353:dbl, "Tolerance Check (T)=Pass.Inlet Temp"=w412:bool, "Tolerance Check (T)=Pass.Tinlet Min"=w393:dbl[], "Tolerance Check (T)=Pass.Tinlet Max"=w392:dbl[], "Data Indexes.Standby Valid"=w330:bool, "Tolerance Check (T)=Pass.Voltage (Heating)"=w342:bool, "Tolerance Check (T)=Pass.Voltage (Min)"=w341:dbl, "Tolerance Check (T)=Pass.Voltage (Max)"=w340:dbl)
          n89 = case shown="False" w404 {
            tunnel: ["False" "True"] -> w403
            frame False {
            }
            frame True {
            }
          }
          n90 = case shown="True" w415 {
            tunnel: ["Out of Specification" "In Specification"] -> w381
            frame False {
            }
            frame True {
            }
          }
          n91 = case shown="True" w414 {
            tunnel: ["Out of Specification" "In Specification"] -> w370
            frame False {
            }
            frame True {
            }
          }
          n92 = case shown="False" w402 {
            tunnel: ["Out of Specification" "In Specification"] -> w400
            frame False {
            }
            frame True {
            }
          }
          n93 = case shown="False" w413 {
            tunnel: ["Out of Specification" "In Specification"] -> w398
            frame False {
            }
            frame True {
            }
          }
          n94 = case shown="False" w366 {
            tunnel: ["Out of Specification" "In Specification"] -> w363
            frame False {
            }
            frame True {
            }
          }
          n95 = case shown="False" w358 {
            tunnel: ["Out of Specification" "In Specification"] -> w361
            frame False {
            }
            frame True {
            }
          }
          n96 = case shown="False" w411 {
            tunnel: ["Out of Specification" "In Specification"] -> w375
            frame False {
            }
            frame True {
            }
          }
          n97 = case shown="False" w354 {
            tunnel: ["Out of Specification" "In Specification"] -> w352
            frame False {
            }
            frame True {
            }
          }
          n98 = case shown="False" w412 {
            tunnel: ["Out of Specification" "In Specification"] -> w389
            frame False {
            }
            frame True {
            }
          }
          n99 = case shown="True" w330 {
            tunnel: ["False" "True"] -> w329
            frame False {
            }
            frame True {
            }
          }
          n100 = case shown="True" w342 {
            tunnel: ["Out of Specification" "In Specification"] -> w345
            frame False {
            }
            frame True {
            }
          }
          n101 = Array Max & Min(array=w393) -> (min value=w391:dbl)  [unwired: 3 out]
          n102 = Array Max & Min(array=w392) -> (max value=w390:dbl)  [unwired: 3 out]
          n103 = Array Max & Min(array=w383) -> (min value=w387:dbl)  [unwired: 3 out]
          n104 = Array Max & Min(array=w382) -> (max value=w386:dbl)  [unwired: 3 out]
          n105 = call "HEWH Add Output Range to Error Code.vi"("Range?"=TRUE, "Units"="V", "Value Max"=w340, "Value Min"=w341, "Input String"=w345) -> ("Display Range"=w339:string)  [unwired: 6 in]
          n106 = call "HEWH Add Output Range to Error Code.vi"("Range?"=TRUE, "Units"="GPM", "Value Max"=w386, "Value Min"=w387, "Input String"=w381) -> ("Display Range"=w380:string)  [unwired: 6 in]
          n107 = call "HEWH Add Output Range to Error Code.vi"("Range?"=FALSE, "Units"="Gal", "Value Min"=w371, "Input String"=w370) -> ("Display Range"=w369:string)  [unwired: 7 in]
          n108 = call "HEWH Add Output Range to Error Code.vi"("Range?"=TRUE, "Units"="°F", "Value Max"=w378, "Value Min"=w379, "Input String"=w398) -> ("Display Range"=w397:string)  [unwired: 6 in]
          n109 = call "HEWH Add Output Range to Error Code.vi"("Range?"=FALSE, "Units"="°F", "Value Min"=w362, "Input String"=w363) -> ("Display Range"=w348:string)  [unwired: 7 in]
          n110 = call "HEWH Add Output Range to Error Code.vi"("Range?"=FALSE, "Units"="°F", "Value Min"=w357, "Input String"=w361) -> ("Display Range"=w347:string)  [unwired: 7 in]
          n111 = call "HEWH Add Output Range to Error Code.vi"("Range?"=TRUE, "Units"="%", "Value Max"=w368, "Value Min"=w367, "Input String"=w375) -> ("Display Range"=w374:string)  [unwired: 6 in]
          n112 = call "HEWH Add Output Range to Error Code.vi"("Range?"=FALSE, "Units"="%", "Value Min"=w353, "Input String"=w352) -> ("Display Range"=w346:string)  [unwired: 7 in]
          n113 = call "HEWH Add Output Range to Error Code.vi"("Range?"=TRUE, "Units"="°F", "Value Max"=w390, "Value Min"=w391, "Input String"=w389) -> ("Display Range"=w388:string)  [unwired: 6 in]
          n114 = Build Array(w338, w337, w336, w335, w334, "Ambient Temperature (67.5°F ±5°F)", "Ambient Temperature On-Time Avg (67.5°F ±1°F)", "Ambient Temperature Off-Time Avg (67.5°F ±2.5°F)", "Ambient Humidity (50% ±5%)", "Ambient Humidity On-Time Avg (50% ±2%)", w333, w331, w332) -> (w408:string[])
          n115 = Build Array(w401, w403, w380, w369, w400, w397, w348, w347, w374, w346, w388, w329, w339) -> (w407:string[])
          n116 = Build Array(w408, w407) -> (w406:string[][])
          n117 = Transpose 2D Array(2D array=w406) -> (transposed array=w405:string[][])
        }
        frame "FHD" {
          n118 = Unbundle By Name(w501) -> ("Tolerance Check (T)=Pass.Data Sheet Check"=w506:string, "Tolerance Check (T)=Pass.Valid Test"=w508:bool, "Tolerance Check (T)=Pass.Flow Rate"=w515:bool, "Tolerance Check (T)=Pass.Flow Rate Min (Tol)"=w487:dbl[], "Tolerance Check (T)=Pass.Flow Rate Max (Tol)"=w486:dbl[], "Tolerance Check (T)=Pass.Ambient Temp (Full Range)"=w514:bool, "Tolerance Check (T)=Pass.Amb Temp Min"=w481:dbl, "Tolerance Check (T)=Pass.Amb Temp Max"=w480:dbl, "Tolerance Check (T)=Pass.Ambient Temp (On-Time AVG)"=w459:bool, "Tolerance Check (T)=Pass.Amb Temp ON Avg"=w457:dbl, "Tolerance Check (T)=Pass.Ambient Temp (Off-Time AVG)"=w458:bool, "Tolerance Check (T)=Pass.Amb Temp OFF Avg"=w456:dbl, "Tolerance Check (T)=Pass.Ambient Humidity (Full Range)"=w512:bool, "Tolerance Check (T)=Pass.Humidity Lower Tolerance (%)"=w477:dbl, "Tolerance Check (T)=Pass.Humidity Upper Tolerance (%)"=w474:dbl, "Tolerance Check (T)=Pass.Ambient Humidity (Runtime)"=w467:bool, "Tolerance Check (T)=Pass.Humidity Avg (Runtime)"=w466:dbl, "Tolerance Check (T)=Pass.Inlet Temp"=w513:bool, "Tolerance Check (T)=Pass.Tinlet Min"=w495:dbl[], "Tolerance Check (T)=Pass.Tinlet Max"=w494:dbl[], "Tolerance Check (T)=Pass.Voltage (Heating)"=w450:bool, "Tolerance Check (T)=Pass.Voltage (Min)"=w449:dbl, "Tolerance Check (T)=Pass.Voltage (Max)"=w448:dbl)
          n119 = case shown="False" w459 {
            tunnel: ["Out of Specification" "In Specification"] -> w465
            frame False {
            }
            frame True {
            }
          }
          n120 = case shown="False" w458 {
            tunnel: ["Out of Specification" "In Specification"] -> w464
            frame False {
            }
            frame True {
            }
          }
          n121 = case shown="True" w512 {
            tunnel: ["Out of Specification" "In Specification"] -> w476
            frame False {
            }
            frame True {
            }
          }
          n122 = case shown="False" w467 {
            tunnel: ["Out of Specification" "In Specification"] -> w470
            frame False {
            }
            frame True {
            }
          }
          n123 = case shown="True" w513 {
            tunnel: ["Out of Specification" "In Specification"] -> w493
            frame False {
            }
            frame True {
            }
          }
          n124 = case shown="True" w508 {
            tunnel: ["False" "True"] -> w507
            frame False {
            }
            frame True {
            }
          }
          n125 = case shown="True" w515 {
            tunnel: ["Out of Specification" "In Specification"] -> w483
            frame False {
            }
            frame True {
            }
          }
          n126 = case shown="True" w514 {
            tunnel: ["Out of Specification" "In Specification"] -> w505
            frame False {
            }
            frame True {
            }
          }
          n127 = Array Max & Min(array=w495) -> (min value=w491:dbl)  [unwired: 3 out]
          n128 = Array Max & Min(array=w494) -> (max value=w490:dbl)  [unwired: 3 out]
          n129 = Array Max & Min(array=w487) -> (min value=w485:dbl)  [unwired: 3 out]
          n130 = Array Max & Min(array=w486) -> (max value=w484:dbl)  [unwired: 3 out]
          n131 = case shown="True" w450 {
            tunnel: ["Out of Specification" "In Specification"] -> w447
            frame False {
            }
            frame True {
            }
          }
          n132 = call "HEWH Add Output Range to Error Code.vi"("Range?"=TRUE, "Units"="V", "Value Max"=w448, "Value Min"=w449, "Input String"=w447) -> ("Display Range"=w446:string)  [unwired: 6 in]
          n133 = call "HEWH Add Output Range to Error Code.vi"("Range?"=TRUE, "Units"="GPM", "Value Max"=w484, "Value Min"=w485, "Input String"=w483) -> ("Display Range"=w482:string)  [unwired: 6 in]
          n134 = call "HEWH Add Output Range to Error Code.vi"("Range?"=TRUE, "Units"="°F", "Value Max"=w480, "Value Min"=w481, "Input String"=w505) -> ("Display Range"=w504:string)  [unwired: 6 in]
          n135 = call "HEWH Add Output Range to Error Code.vi"("Range?"=FALSE, "Units"="°F", "Value Min"=w457, "Input String"=w465) -> ("Display Range"=w455:string)  [unwired: 7 in]
          n136 = call "HEWH Add Output Range to Error Code.vi"("Range?"=FALSE, "Units"="°F", "Value Min"=w456, "Input String"=w464) -> ("Display Range"=w454:string)  [unwired: 7 in]
          n137 = call "HEWH Add Output Range to Error Code.vi"("Range?"=TRUE, "Units"="%", "Value Max"=w474, "Value Min"=w477, "Input String"=w476) -> ("Display Range"=w475:string)  [unwired: 6 in]
          n138 = call "HEWH Add Output Range to Error Code.vi"("Range?"=FALSE, "Units"="%", "Value Min"=w466, "Input String"=w470) -> ("Display Range"=w453:string)  [unwired: 7 in]
          n139 = call "HEWH Add Output Range to Error Code.vi"("Range?"=TRUE, "Units"="°F", "Value Max"=w490, "Value Min"=w491, "Input String"=w493) -> ("Display Range"=w492:string)  [unwired: 6 in]
          n140 = Build Array(w506, w507, w482, w504, w455, w454, w475, w453, w492, w446) -> (w510:string[])
          n141 = Build Array(w445, w444, w443, "Ambient Temperature (67.5°F ±5°F)", "Ambient Temperature On-Time Avg (67.5°F ±1°F)", "Ambient Temperature Off-Time Avg (67.5°F ±2.5°F)", "Ambient Humidity (50% ±5%)", "Ambient Humidity On-Time Avg (50% ±2%)", w442, w441) -> (w511:string[])
          n142 = Build Array(w511, w510) -> (w509:string[][])
          n143 = Transpose 2D Array(2D array=w509) -> (transposed array=w500:string[][])
        }
      }
    }
    frame "Gas Storage (Non-Electric)" {
      n144 = case shown="\"FHD\"" w542 {
        tunnel: w544 -> [w595 w638]
        tunnel: [w587 w637] -> w543
        tunnel: w541 -> [w554 w614]
        tunnel: w540 -> [w553 w613]
        tunnel: w539 -> [w552 w612]
        tunnel: w538 -> [w551 _]
        tunnel: w537 -> [w550 _]
        tunnel: w536 -> [w549 w611]
        tunnel: w535 -> [w548 w610]
        tunnel: w534 -> [w547 _]
        frame "UEF", Default {
          n145 = Unbundle By Name(w595) -> ("Tolerance Check (T)=Pass.Data Sheet Check"=w584:string, "Tolerance Check (T)=Pass.Valid Test"=w586:bool, "Tolerance Check (T)=Pass.Flow Rate"=w594:bool, "Tolerance Check (T)=Pass.Flow Rate Min (Tol)"=w561:dbl[], "Tolerance Check (T)=Pass.Flow Rate Max (Tol)"=w560:dbl[], "Tolerance Check (T)=Pass.Totalized Flow"=w593:bool, "Tolerance Check (T)=Pass.Total Volume Tolerance (Gal)"=w555:dbl, "Tolerance Check (T)=Pass.Individual Totalized Flow"=w582:bool, "Tolerance Check (T)=Pass.Ambient Temp (Full Range)"=w592:bool, "Tolerance Check (T)=Pass.Amb Temp Min"=w577:dbl, "Tolerance Check (T)=Pass.Amb Temp Max"=w576:dbl, "Tolerance Check (T)=Pass.Inlet Temp"=w591:bool, "Tolerance Check (T)=Pass.Tinlet Min"=w571:dbl[], "Tolerance Check (T)=Pass.Tinlet Max"=w570:dbl[], "Data Indexes.Standby Valid"=w546:bool)
          n146 = case shown="True" w592 {
            tunnel: ["Out of Specification" "In Specification"] -> w579
            frame False {
            }
            frame True {
            }
          }
          n147 = case shown="True" w582 {
            tunnel: ["Out of Specification" "In Specification"] -> w583
            frame False {
            }
            frame True {
            }
          }
          n148 = case shown="True" w586 {
            tunnel: ["False" "True"] -> w585
            frame False {
            }
            frame True {
            }
          }
          n149 = case shown="True" w594 {
            tunnel: ["Out of Specification" "In Specification"] -> w563
            frame False {
            }
            frame True {
            }
          }
          n150 = case shown="True" w593 {
            tunnel: ["Out of Specification" "In Specification"] -> w557
            frame False {
            }
            frame True {
            }
          }
          n151 = case shown="True" w591 {
            tunnel: ["Out of Specification" "In Specification"] -> w569
            frame False {
            }
            frame True {
            }
          }
          n152 = case shown="True" w546 {
            tunnel: ["False" "True"] -> w545
            frame False {
            }
            frame True {
            }
          }
          n153 = Array Max & Min(array=w561) -> (min value=w567:dbl)  [unwired: 3 out]
          n154 = Array Max & Min(array=w560) -> (max value=w566:dbl)  [unwired: 3 out]
          n155 = Array Max & Min(array=w571) -> (min value=w575:dbl)  [unwired: 3 out]
          n156 = Array Max & Min(array=w570) -> (max value=w574:dbl)  [unwired: 3 out]
          n157 = Build Array(w554, w553, w552, w551, w550, w549, w548, w547) -> (w590:string[])
          n158 = call "HEWH Add Output Range to Error Code.vi"("Range?"=TRUE, "Units"="GPM", "Value Max"=w566, "Value Min"=w567, "Input String"=w563) -> ("Display Range"=w562:string)  [unwired: 6 in]
          n159 = call "HEWH Add Output Range to Error Code.vi"("Range?"=FALSE, "Units"="Gal", "Value Min"=w555, "Input String"=w557) -> ("Display Range"=w556:string)  [unwired: 7 in]
          n160 = call "HEWH Add Output Range to Error Code.vi"("Range?"=TRUE, "Units"="°F", "Value Max"=w576, "Value Min"=w577, "Input String"=w579) -> ("Display Range"=w578:string)  [unwired: 6 in]
          n161 = call "HEWH Add Output Range to Error Code.vi"("Range?"=TRUE, "Units"="°F", "Value Max"=w574, "Value Min"=w575, "Input String"=w569) -> ("Display Range"=w568:string)  [unwired: 6 in]
          n162 = Build Array(w584, w585, w562, w556, w583, w578, w568, w545) -> (w589:string[])
          n163 = Build Array(w590, w589) -> (w588:string[][])
          n164 = Transpose 2D Array(2D array=w588) -> (transposed array=w587:string[][])
        }
        frame "FHD" {
          n165 = Unbundle By Name(w638) -> ("Tolerance Check (T)=Pass.Data Sheet Check"=w639:string, "Tolerance Check (T)=Pass.Valid Test"=w641:bool, "Tolerance Check (T)=Pass.Flow Rate"=w647:bool, "Tolerance Check (T)=Pass.Flow Rate Min (Tol)"=w618:dbl[], "Tolerance Check (T)=Pass.Flow Rate Max (Tol)"=w617:dbl[], "Tolerance Check (T)=Pass.Ambient Temp (Full Range)"=w646:bool, "Tolerance Check (T)=Pass.Amb Temp Min"=w632:dbl, "Tolerance Check (T)=Pass.Amb Temp Max"=w631:dbl, "Tolerance Check (T)=Pass.Inlet Temp"=w645:bool, "Tolerance Check (T)=Pass.Tinlet Min"=w624:dbl[], "Tolerance Check (T)=Pass.Tinlet Max"=w623:dbl[])
          n166 = case shown="True" w641 {
            tunnel: ["False" "True"] -> w640
            frame False {
            }
            frame True {
            }
          }
          n167 = case shown="True" w647 {
            tunnel: ["Out of Specification" "In Specification"] -> w616
            frame False {
            }
            frame True {
            }
          }
          n168 = case shown="True" w646 {
            tunnel: ["Out of Specification" "In Specification"] -> w634
            frame False {
            }
            frame True {
            }
          }
          n169 = case shown="True" w645 {
            tunnel: ["Out of Specification" "In Specification"] -> w626
            frame False {
            }
            frame True {
            }
          }
          n170 = Array Max & Min(array=w618) -> (min value=w622:dbl)  [unwired: 3 out]
          n171 = Array Max & Min(array=w617) -> (max value=w621:dbl)  [unwired: 3 out]
          n172 = Array Max & Min(array=w624) -> (min value=w630:dbl)  [unwired: 3 out]
          n173 = Array Max & Min(array=w623) -> (max value=w629:dbl)  [unwired: 3 out]
          n174 = call "HEWH Add Output Range to Error Code.vi"("Range?"=TRUE, "Units"="GPM", "Value Max"=w621, "Value Min"=w622, "Input String"=w616) -> ("Display Range"=w615:string)  [unwired: 6 in]
          n175 = call "HEWH Add Output Range to Error Code.vi"("Range?"=TRUE, "Units"="°F", "Value Max"=w631, "Value Min"=w632, "Input String"=w634) -> ("Display Range"=w633:string)  [unwired: 6 in]
          n176 = call "HEWH Add Output Range to Error Code.vi"("Range?"=TRUE, "Units"="°F", "Value Max"=w629, "Value Min"=w630, "Input String"=w626) -> ("Display Range"=w625:string)  [unwired: 6 in]
          n177 = Build Array(w614, w613, w612, w611, w610) -> (w644:string[])
          n178 = Build Array(w639, w640, w615, w633, w625) -> (w643:string[])
          n179 = Build Array(w644, w643) -> (w642:string[][])
          n180 = Transpose 2D Array(2D array=w642) -> (transposed array=w637:string[][])
        }
      }
    }
  }
  n181 = Build Array (concatenate)(w8, w5, w4) -> (w3:string[][])
  n182 = Build Array (concatenate)(w7, w5, w4) -> (w2:string[][])
  n183 = Bundle By Name(cluster="UEF Calculated Values Input", "Test Information.UEF Report Information"=w3, "Test Information.FHR Report Information"=w2) -> (→"UEF Calculated Values Output":T2)
  "error out" <- "error in (no error)"
